vi "Dielectric vs Temperature - freq (4284A).vi"() -> ()   [LabVIEW 2010]
uses:
  <vilib>/Instr/_visa.llb/VISA Configure Serial Port (Instr).vi
  Instance          14 32Saved   K vs Temp - freq (4284A) .vi
  Instance          13 32Saved   K vs Temp - freq (4284A) .vi
  Instance          12 32Saved   K vs Temp - freq (4284A) .vi
  Instance          11 32Saved   K vs Temp - freq (4284A) .vi
  Instance          26 32Saved   K vs Temp - freq (4284A) .vi
  Instance          25 32Saved   K vs Temp - freq (4284A) .vi
  Instance          10 32Saved   K vs Temp - freq (4284A) .vi
  Instance           9 32Saved   K vs Temp - freq (4284A) .vi
  Instance           8 32Saved   K vs Temp - freq (4284A) .vi
  Instance           7 32Saved   K vs Temp - freq (4284A) .vi
  Instance          24 32Saved   K vs Temp - freq (4284A) .vi
  Instance          22 32Saved   K vs Temp - freq (4284A) .vi
  Instance          20 32Saved   K vs Temp - freq (4284A) .vi
  Instance          18 32Saved   K vs Temp - freq (4284A) .vi
  Instance          23 32Saved   K vs Temp - freq (4284A) .vi
  Instance          21 32Saved   K vs Temp - freq (4284A) .vi
  Instance          19 32Saved   K vs Temp - freq (4284A) .vi
  Instance          17 32Saved   K vs Temp - freq (4284A) .vi
  Instance          16 32Saved   K vs Temp - freq (4284A) .vi
  Instance          15 32Saved   K vs Temp - freq (4284A) .vi
  Instance           6 32Saved   K vs Temp - freq (4284A) .vi
  Instance           5 32Saved   K vs Temp - freq (4284A) .vi
  <vilib>/Utility/file.llb/Write To Spreadsheet File (DBL).vi
panel:
  in  "Freq Value (Hz) (1MHz)":dbl=1000000.0
  out "tand1M":dbl
  out "K1M":dbl
  out "C1M":dbl
  out "Temp1MHz":dbl format="%#_3g"
  in  "Freq Value (Hz) (500kHz)":dbl=500000.0
  out "tand500k":dbl
  out "K500k":dbl
  out "C500k":dbl
  out "Temp500kHz":dbl format="%#_3g"
  in  "Freq Value (Hz) (250kHz)":dbl=250000.0
  out "tand250k":dbl
  out "K250k":dbl
  out "C250k":dbl
  out "Temp250kHz":dbl format="%#_3g"
  in  "Freq Value (Hz) (100kHz)":dbl=100000.0
  out "tand100k":dbl
  out "K100k":dbl
  out "C100k":dbl
  out "Temp100kHz":dbl format="%#_3g"
  in  "Freq Value (Hz) (50kHz)":dbl=50000.0
  out "tand50k":dbl
  out "K50k":dbl
  out "C50k":dbl
  out "Temp50kHz":dbl format="%#_3g"
  in  "Freq Value (Hz) (25kHz)":dbl=25000.0
  out "tand25k":dbl
  out "K25k":dbl
  out "C25k":dbl
  out "Temp25kHz":dbl format="%#_3g"
  in  "Freq Value (Hz) (10kHz)":dbl=10000.0
  out "tand10k":dbl
  out "K10k":dbl
  out "C10k":dbl
  out "Temp10kHz":dbl format="%#_3g"
  in  "Freq Value (Hz) (5kHz)":dbl=5000.0
  out "tand5k":dbl
  out "K5k":dbl
  out "C5k":dbl
  out "Temp5kHz":dbl format="%#_3g"
  in  "Freq Value (Hz) (2.5kHz)":dbl=2500.0
  out "tand2.5k":dbl
  out "K2.5k":dbl
  out "C2.5k":dbl
  out "Temp2.5kHz":dbl format="%#_3g"
  in  "Freq Value (Hz) (1kHz)":dbl=1000.0
  out "tand1k":dbl
  out "K1k":dbl
  out "C1k":dbl
  out "Temp1kHz":dbl format="%#_3g"
  in  "tand500k":dbl[](array[numeric])
  in  "K500k":dbl[](array[numeric])
  in  "Temp500k":dbl[](array[numeric])
  out "Temp500Hz":dbl format="%#_3g"
  out "C500":dbl
  out "?":dbl
  out "tand500":dbl
  in  "Freq Value (Hz) (500Hz)":dbl=500.0
  in  "Freq Value (Hz) (250Hz)":dbl=250.0
  in  "Freq Value (Hz) (100Hz)":dbl=100.0
  in  "Freq Value (Hz) (50Hz)":dbl=50.0
  in  "Freq Value (Hz) (25Hz)":dbl=25.0
  in  "tand100k":dbl[](array[numeric])
  in  "tand10k":dbl[](array[numeric])
  in  "tand1k":dbl[](array[numeric])
  in  "tand100":dbl[](array[numeric])
  in  "K100k":dbl[](array[numeric])
  in  "K10k":dbl[](array[numeric])
  in  "K1k":dbl[](array[numeric])
  in  "K100":dbl[](array[numeric])
  in  "Temp100k":dbl[](array[numeric])
  in  "Temp10k":dbl[](array[numeric])
  in  "Temp1k":dbl[](array[numeric])
  in  "Temp100":dbl[](array[numeric])
  out "Temp250Hz":dbl format="%#_3g"
  out "Temp100Hz":dbl format="%#_3g"
  out "tand25":dbl
  out "Temp50Hz":dbl format="%#_3g"
  in  "VISA Omega (Serial - COM1)":refnum<visa-resource-name>
  in  "VISA Agilent 4284A (GPIB)":refnum<visa-resource-name>
  in  "Run":bool
  out "Thickness":dbl
  out "Area":dbl
  in  "stop":bool
  out "tand250":dbl
  out "tand100":dbl
  out "tand50":dbl
  out "K250":dbl
  out "K100":dbl
  out "K50":dbl
  out "K25":dbl
  out "C250":dbl
  out "C100":dbl
  out "C50":dbl
  out "C25":dbl
  out "Temp25Hz":dbl format="%#_3g"
  out "Dielectric Loss vs. Temperature":cluster{"Y":dbl[], "Y":dbl[]}[](graph)
  out "Relative Permittivity vs. Temperature":cluster{"Y":dbl[], "Y":dbl[]}[](graph)
  in  "Comment (Sample's Name, compositions, whatever you want,..)":string
  in  "Thickness (mm)":dbl
  in  "Diameter (mm)":dbl
  in  "Path & File Name (*.txt)":path
  # "Temperature (C)"
  # "Frequency (Hz)"
  # "Capacitance (F)"
  # "Relative Permittivity"
  # "Dielectric Loss"
  # "Sample Details"
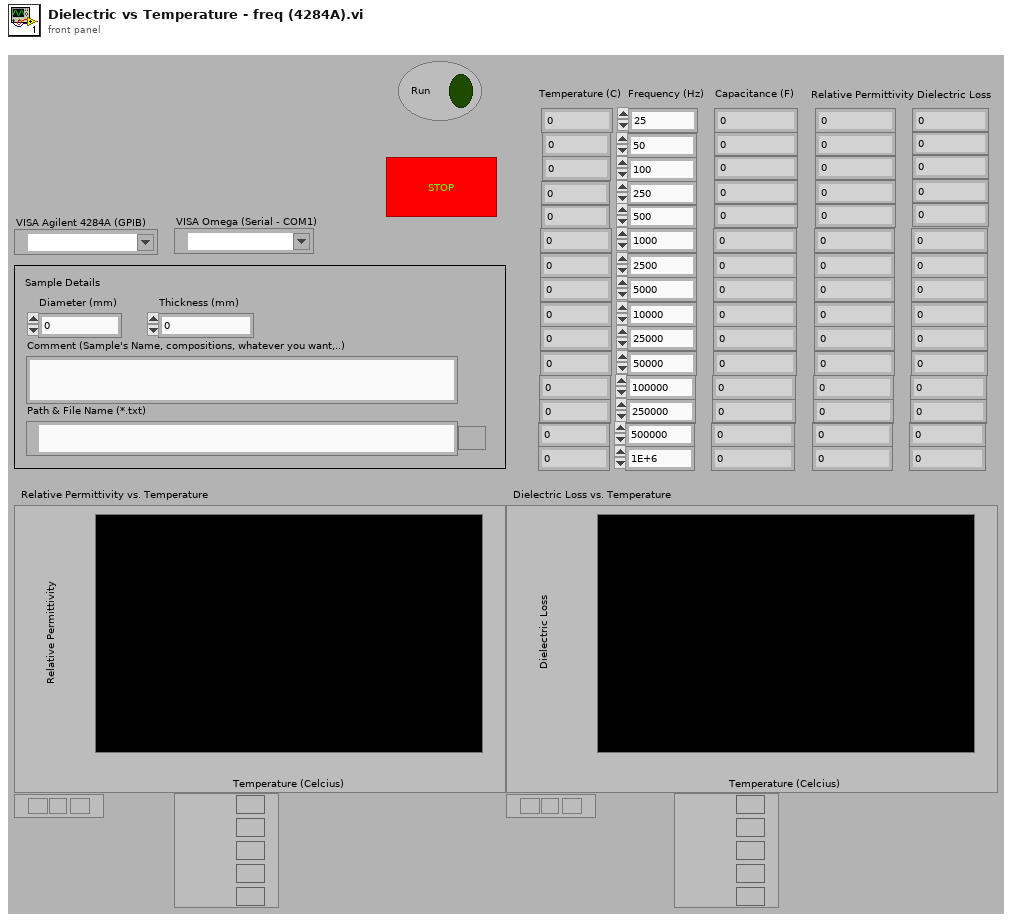
[diagram p1: front panel]
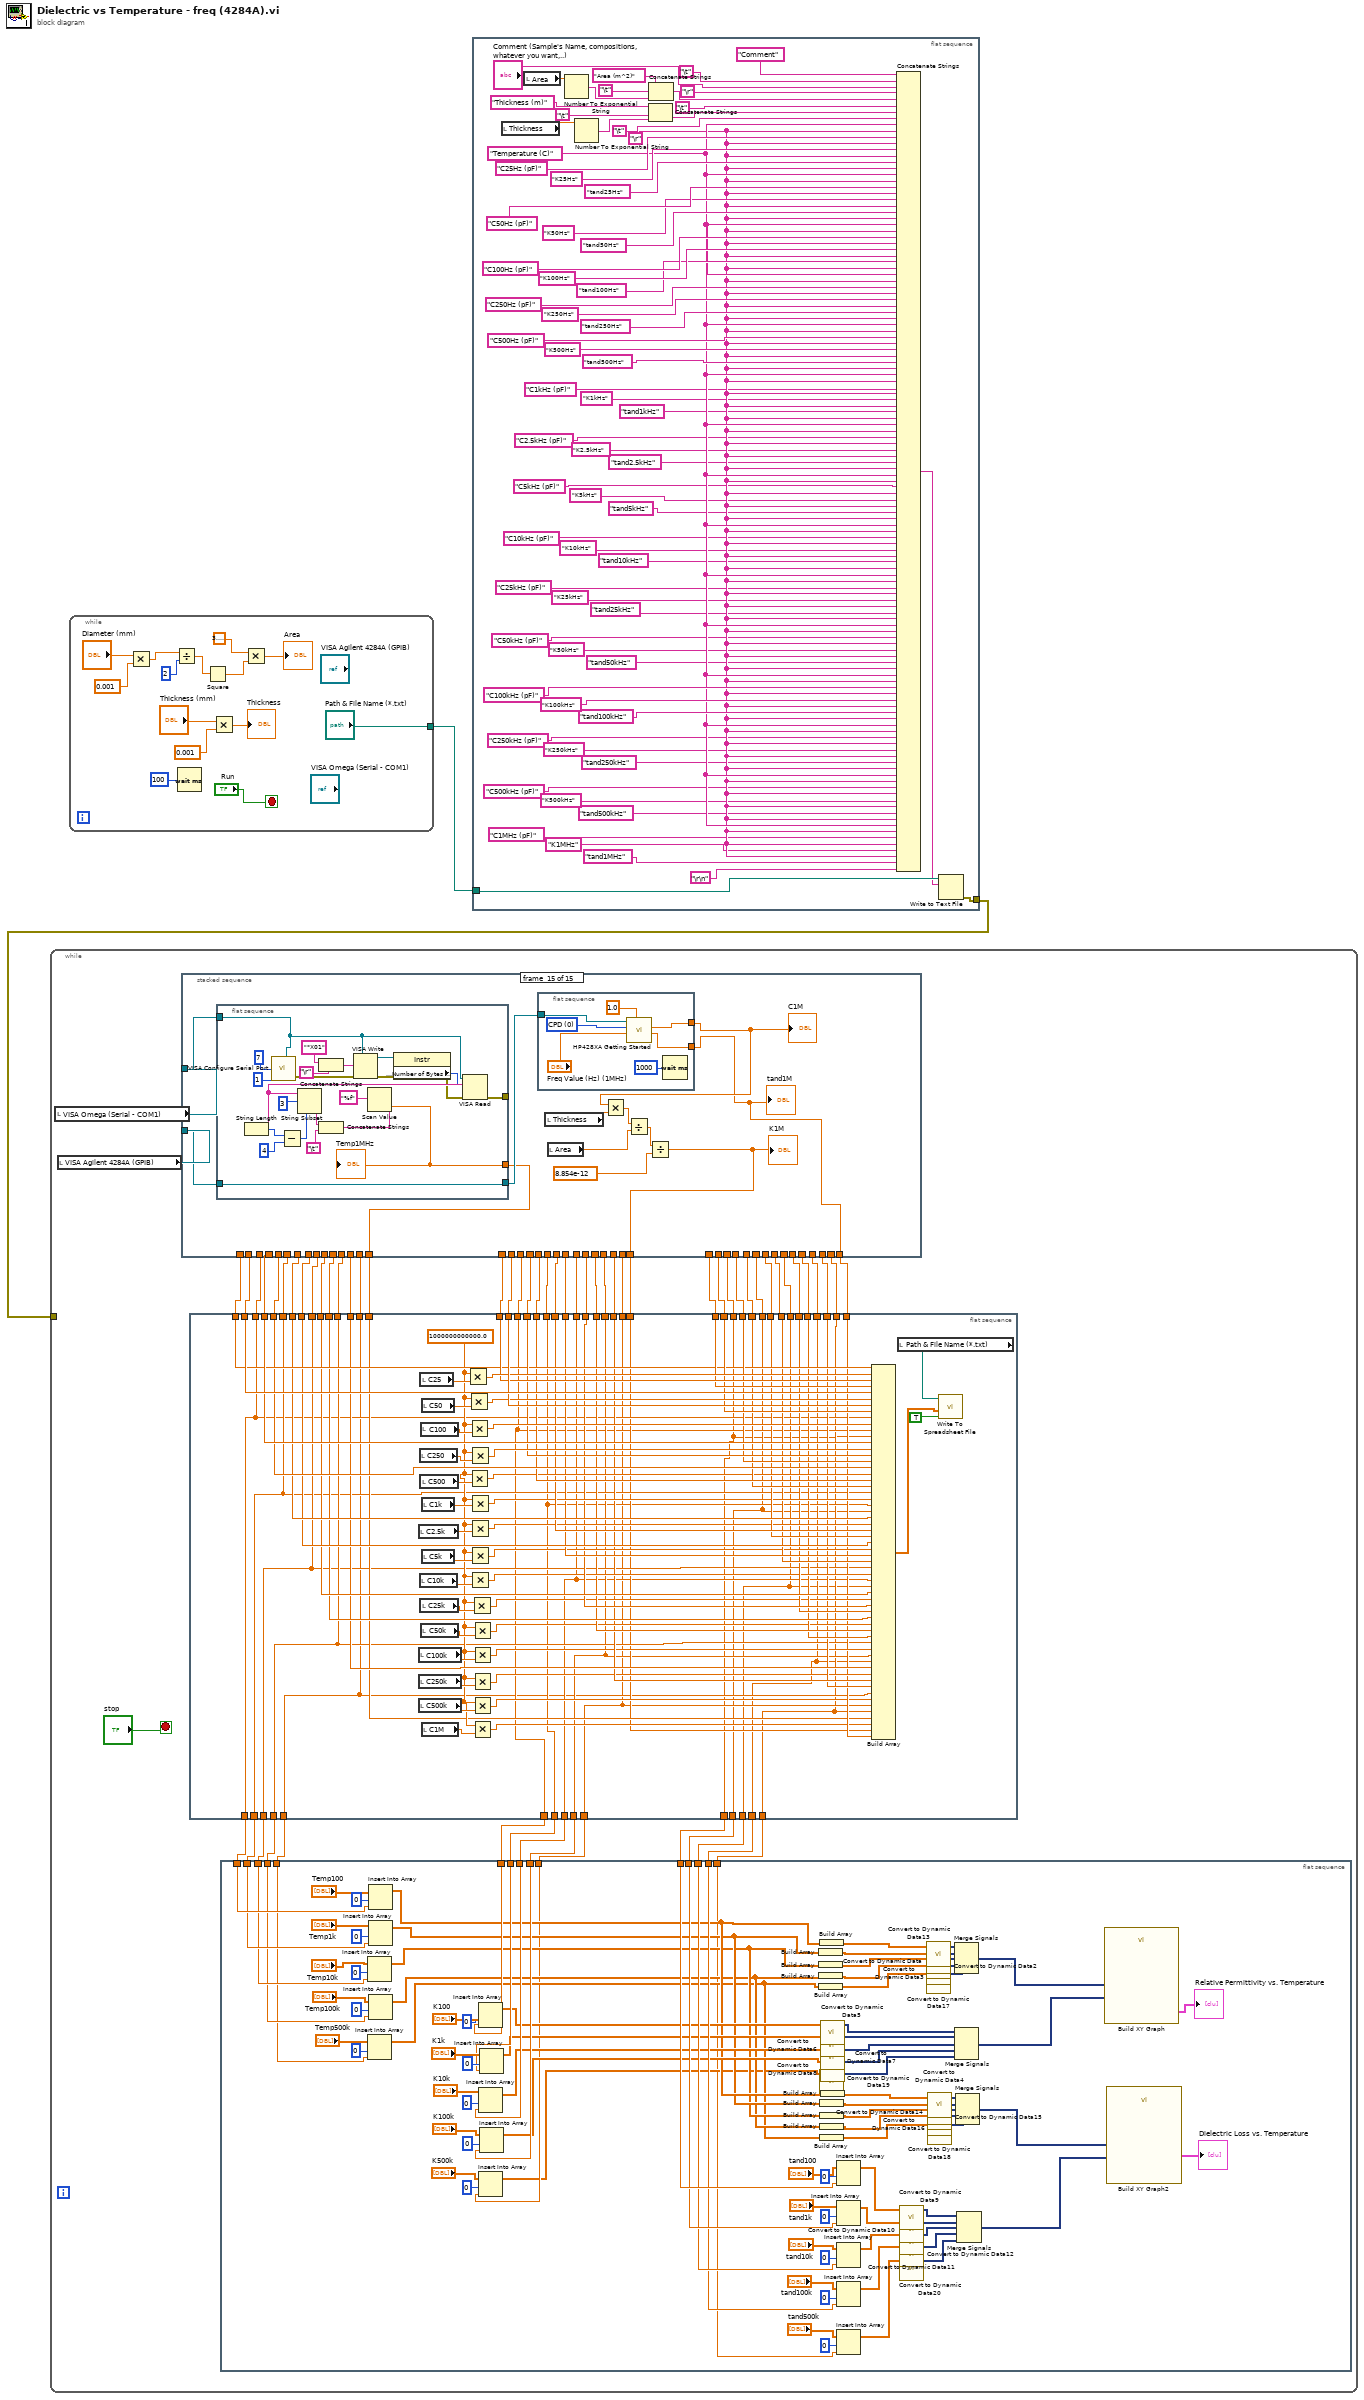
[diagram p0: block diagram]
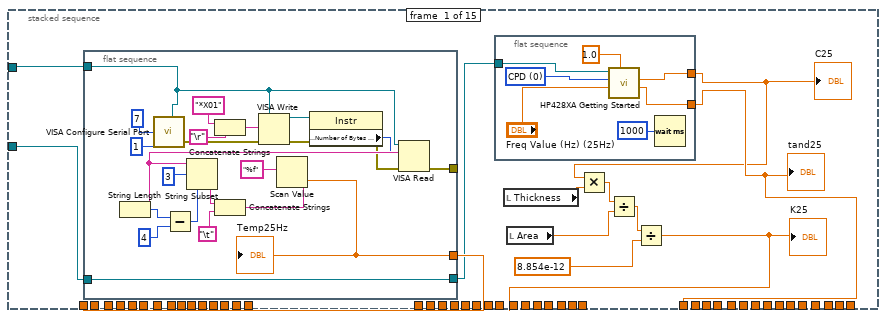
[diagram p2: hidden frame]
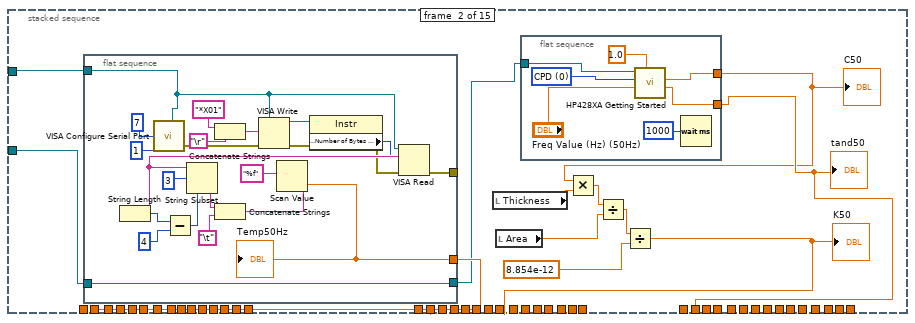
[diagram p3: hidden frame]
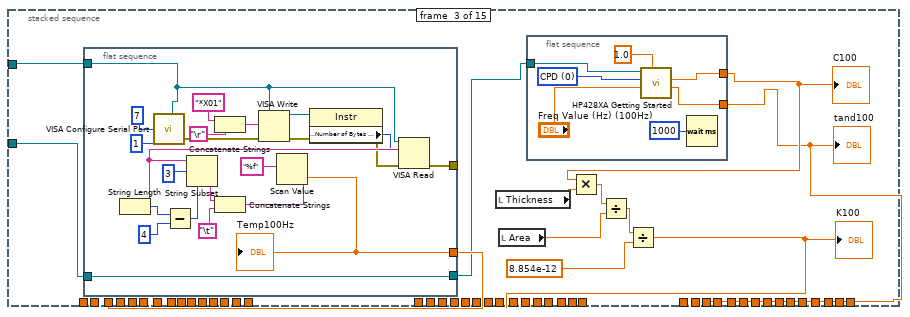
[diagram p4: hidden frame]
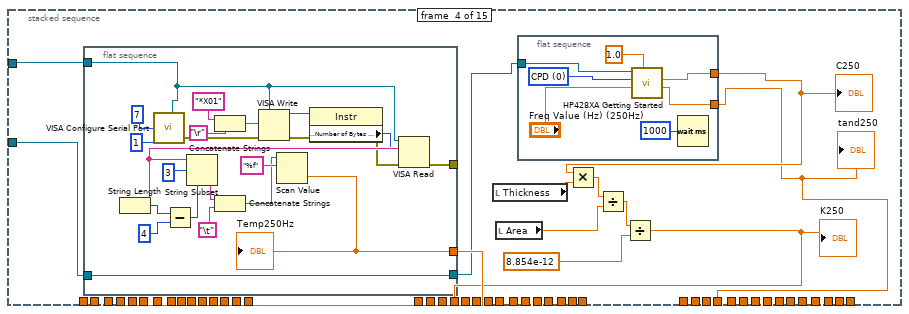
[diagram p5: hidden frame]
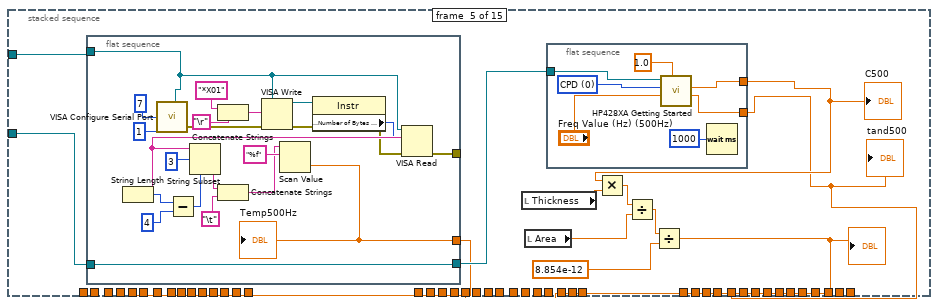
[diagram p6: hidden frame]
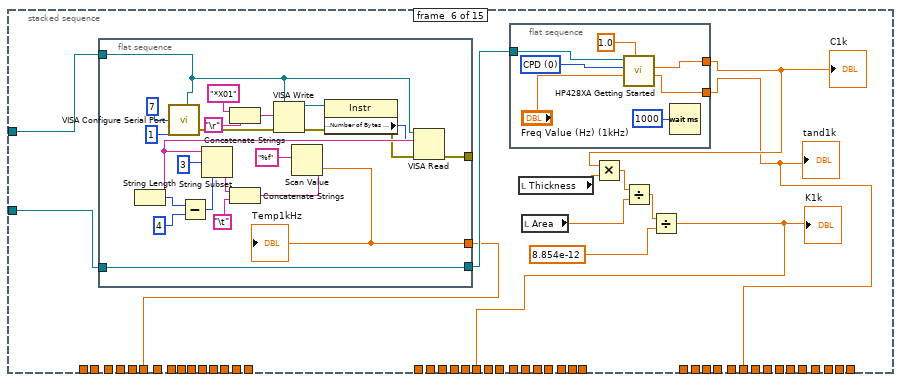
[diagram p7: hidden frame]
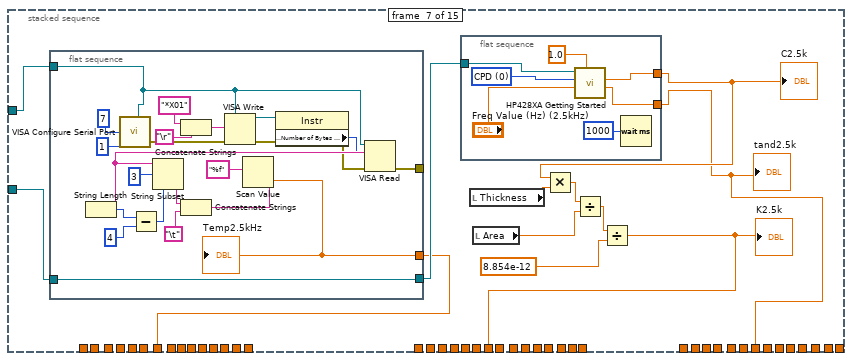
[diagram p8: hidden frame]
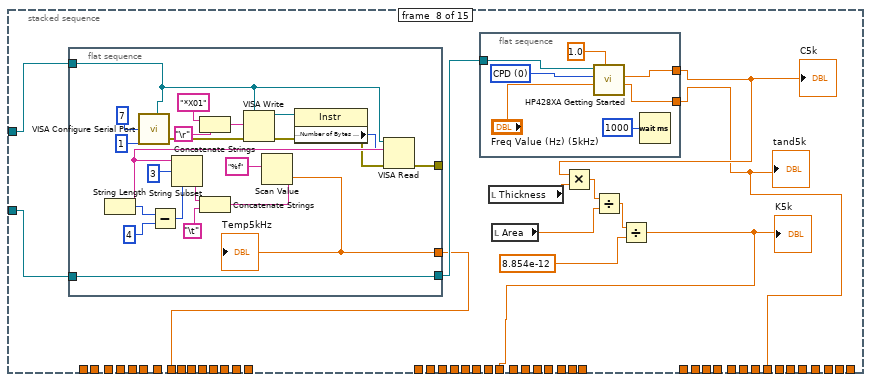
[diagram p9: hidden frame]
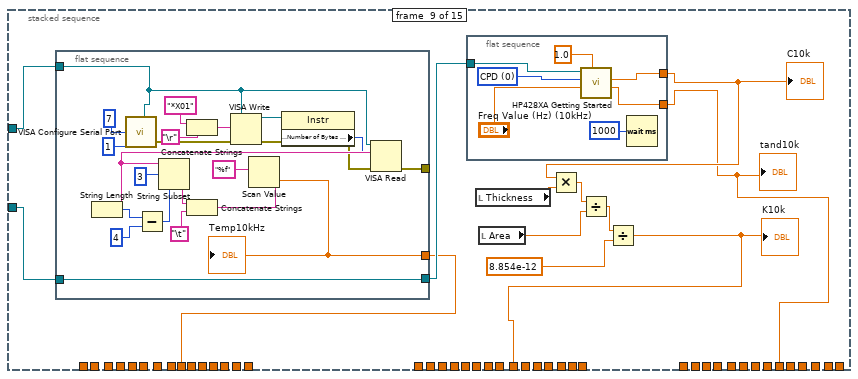
[diagram p10: hidden frame]
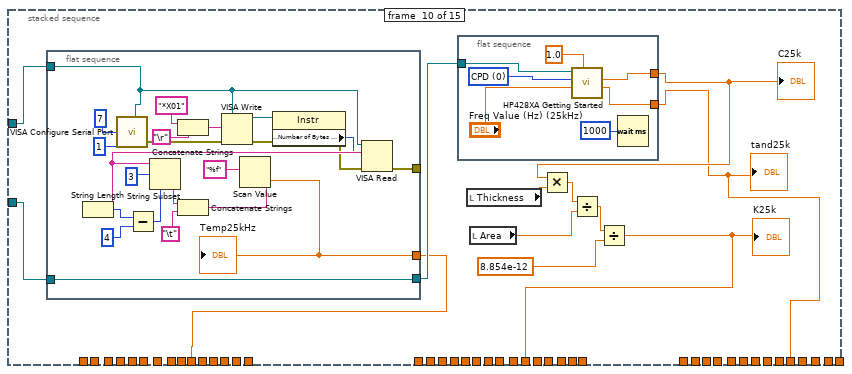
[diagram p11: hidden frame]
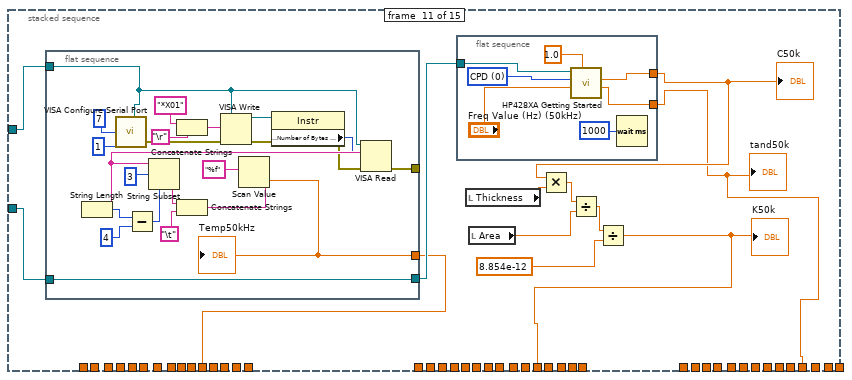
[diagram p12: hidden frame]
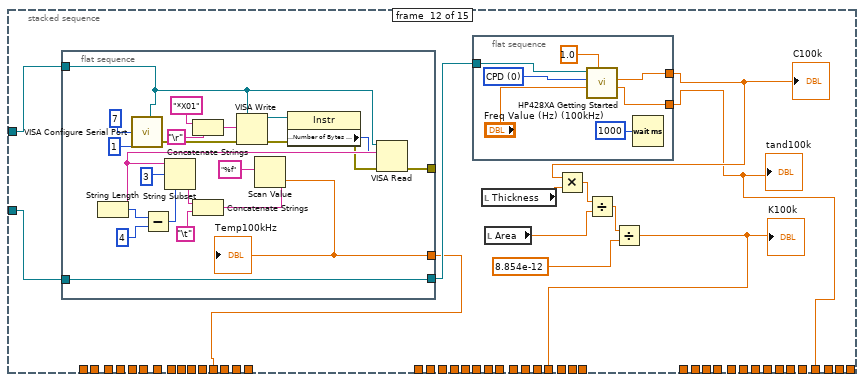
[diagram p13: hidden frame]
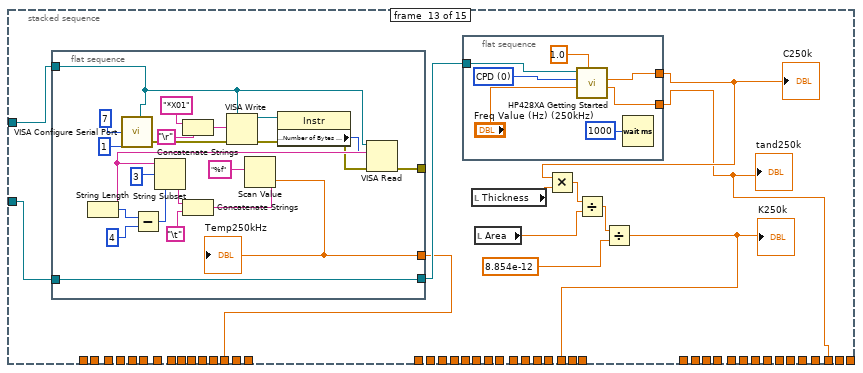
[diagram p14: hidden frame]
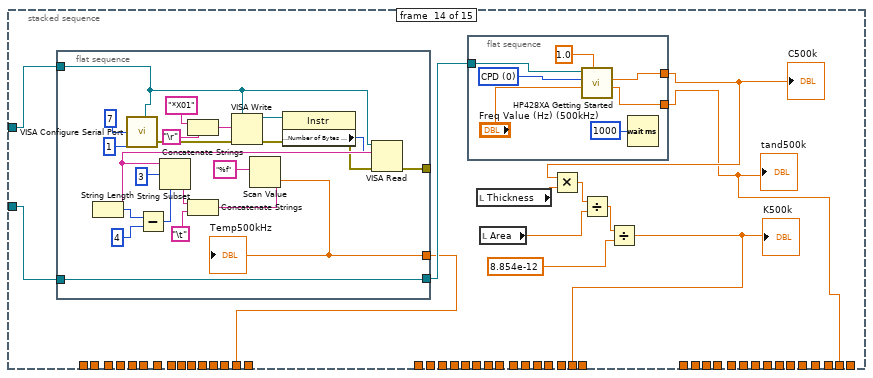
[diagram p15: hidden frame]
diagram:
  n1 = while {
    tunnel: w1 -> [_]
    stop <- "stop" stop-if-true
    n2 = local read "VISA Omega (Serial - COM1)"() -> (w52:refnum<visa-resource-name>)
    n3 = local read "VISA Agilent 4284A (GPIB)"() -> (w51:refnum<visa-resource-name>)
    n4 = stacked-sequence {
      tunnel: w52 -> [w252 w294 w336 w378 w413 w455 w497 w539 w581 w623 w665 w707 w749 w791 w833]
      tunnel: w51 -> [w251 w293 w335 w377 w414 w454 w496 w538 w580 w622 w664 w706 w748 w790 w832]
      tunnel: [w245 _ _ _ _ _ _ _ _ _ _ _ _ _ _] -> w53
      tunnel: [_ w287 _ _ _ _ _ _ _ _ _ _ _ _ _] -> w64
      tunnel: [_ _ w329 _ _ _ _ _ _ _ _ _ _ _ _] -> w63
      tunnel: [_ _ _ w371 _ _ _ _ _ _ _ _ _ _ _] -> w62
      tunnel: [w244 _ _ _ _ _ _ _ _ _ _ _ _ _ _] -> w61
      tunnel: [_ w286 _ _ _ _ _ _ _ _ _ _ _ _ _] -> w60
      tunnel: [_ _ w328 _ _ _ _ _ _ _ _ _ _ _ _] -> w59
      tunnel: [_ _ _ w370 _ _ _ _ _ _ _ _ _ _ _] -> w58
      tunnel: [w242 _ _ _ _ _ _ _ _ _ _ _ _ _ _] -> w57
      tunnel: [_ w285 _ _ _ _ _ _ _ _ _ _ _ _ _] -> w56
      tunnel: [_ _ w325 _ _ _ _ _ _ _ _ _ _ _ _] -> w55
      tunnel: [_ _ _ w367 _ _ _ _ _ _ _ _ _ _ _] -> w54
      tunnel: [_ _ _ _ w411 _ _ _ _ _ _ _ _ _ _] -> w50
      tunnel: [_ _ _ _ w410 _ _ _ _ _ _ _ _ _ _] -> w49
      tunnel: [_ _ _ _ w409 _ _ _ _ _ _ _ _ _ _] -> w48
      tunnel: [_ _ _ _ _ w453 _ _ _ _ _ _ _ _ _] -> w47
      tunnel: [_ _ _ _ _ w452 _ _ _ _ _ _ _ _ _] -> w46
      tunnel: [_ _ _ _ _ w451 _ _ _ _ _ _ _ _ _] -> w45
      tunnel: [_ _ _ _ _ _ w495 _ _ _ _ _ _ _ _] -> w44
      tunnel: [_ _ _ _ _ _ w494 _ _ _ _ _ _ _ _] -> w43
      tunnel: [_ _ _ _ _ _ w493 _ _ _ _ _ _ _ _] -> w42
      tunnel: [_ _ _ _ _ _ _ w537 _ _ _ _ _ _ _] -> w41
      tunnel: [_ _ _ _ _ _ _ w536 _ _ _ _ _ _ _] -> w40
      tunnel: [_ _ _ _ _ _ _ w535 _ _ _ _ _ _ _] -> w39
      tunnel: [_ _ _ _ _ _ _ _ w579 _ _ _ _ _ _] -> w38
      tunnel: [_ _ _ _ _ _ _ _ w578 _ _ _ _ _ _] -> w37
      tunnel: [_ _ _ _ _ _ _ _ w577 _ _ _ _ _ _] -> w36
      tunnel: [_ _ _ _ _ _ _ _ _ w621 _ _ _ _ _] -> w35
      tunnel: [_ _ _ _ _ _ _ _ _ w620 _ _ _ _ _] -> w34
      tunnel: [_ _ _ _ _ _ _ _ _ w619 _ _ _ _ _] -> w33
      tunnel: [_ _ _ _ _ _ _ _ _ _ w663 _ _ _ _] -> w32
      tunnel: [_ _ _ _ _ _ _ _ _ _ w662 _ _ _ _] -> w31
      tunnel: [_ _ _ _ _ _ _ _ _ _ w661 _ _ _ _] -> w30
      tunnel: [_ _ _ _ _ _ _ _ _ _ _ w705 _ _ _] -> w29
      tunnel: [_ _ _ _ _ _ _ _ _ _ _ w704 _ _ _] -> w28
      tunnel: [_ _ _ _ _ _ _ _ _ _ _ w703 _ _ _] -> w27
      tunnel: [_ _ _ _ _ _ _ _ _ _ _ _ w747 _ _] -> w26
      tunnel: [_ _ _ _ _ _ _ _ _ _ _ _ w746 _ _] -> w25
      tunnel: [_ _ _ _ _ _ _ _ _ _ _ _ w745 _ _] -> w24
      tunnel: [_ _ _ _ _ _ _ _ _ _ _ _ _ w789 _] -> w23
      tunnel: [_ _ _ _ _ _ _ _ _ _ _ _ _ w788 _] -> w22
      tunnel: [_ _ _ _ _ _ _ _ _ _ _ _ _ w787 _] -> w21
      tunnel: [_ _ _ _ _ _ _ _ _ _ _ _ _ _ w831] -> w18
      tunnel: [_ _ _ _ _ _ _ _ _ _ _ _ _ _ w830] -> w19
      tunnel: [_ _ _ _ _ _ _ _ _ _ _ _ _ _ w829] -> w20
      frame #0 {
        n5 = flat-sequence {
          tunnel: w252 -> [w263]
          tunnel: [w262] -> _
          tunnel: [w261] -> w245
          tunnel: w251 -> [w260]
          tunnel: [w260] -> w243
          frame #0 {
            n6 = call-poly "VISA Configure Serial Port"("VISA resource name"=w263, "data bits (8)"=7, "parity (0:none)"=1) -> ("error out"=w268:errorcluster)  [unwired: 11 in, 1 out]
            n7 = Concatenate Strings("*X01", "\r") -> (w271:string)
            n8 = VISA Write(VISA resource name=w263, write buffer=w271, error in (no error)=w268) -> (VISA resource name out=w282:refnum<visa-resource-name>, error out=w272:errorcluster)  [unwired: 1 out]
            n9 = property class="Instr"(reference=w282, error in=w272) -> (error out=w273:errorcluster, "Serial Settings:Number of Bytes at Serial Port"=w274:u32)  [unwired: 1 out]
            n10 = VISA Read(VISA resource name=w263, byte count=w274, error in (no error)=w273) -> (read buffer=w275:string, error out=w262:errorcluster)  [unwired: 2 out]
            n11 = String Length(string=w275) -> (length=w277:i32)
            n12 = Subtract(x=w277, y=4) -> (x-y=w279:i32)
            n13 = String Subset(string=w275, offset (0)=3, length (rest)=w279) -> (substring=w280:string)
            n14 = Concatenate Strings(w280, "\t") -> (w264:string)
            n15 = Scan Value(string=w264, format string="%f") -> (value=w261:dbl)  [unwired: 1 in, 1 out]
            "Temp25Hz" <- w261
          }
        }
        n16 = flat-sequence {
          tunnel: w243 -> [w258]
          tunnel: [w255] -> w242
          tunnel: [w254] -> w241
          frame #0 {
            w257 = u32 0 items=["CPD", "CPQ", "CPG", "CPRP", "CSD", "CSQ", "CSRS", "LPQ", "LPD", "LPG", "LPRP", "LSD", "LSQ", "LSRS", "RX", "ZTD", "ZTR", "GB", "YTD", "YTR"] ("Imp Type (0: CPD)")
            n17 = call "HP428XA Getting Started.vi"("Voltage Level (V) (1.0V)"=1.0, "Freq Value (Hz) (1.0 MHz)"="Freq Value (Hz) (25Hz)", "Imp Type (0: CPD)"=w257, "GPIB Address (15)"=w258) -> ("Secondary Value"=w255:dbl, "Primary Value"=w254:dbl)  [unwired: 4 in, 2 out]
            n18 = Wait (ms)(milliseconds to wait=u32 1000) -> ()  [unwired: 1 out]
          }
        }
        n19 = local read "Thickness"() -> (w250:dbl)
        n20 = local read "Area"() -> (w248:dbl)
        n21 = Multiply(x=w241, y=w250) -> (x*y=w249:dbl)
        n22 = Divide(x=w249, y=w248) -> (x/y=w247:dbl)
        n23 = Divide(x=w247, y=8.854e-12) -> (x/y=w244:dbl)
        "K25" <- w244
        "C25" <- w241
        "tand25" <- w242
      }
      frame #1 {
        n24 = flat-sequence {
          tunnel: w294 -> [w305]
          tunnel: [w304] -> _
          tunnel: [w303] -> w287
          tunnel: w293 -> [w302]
          tunnel: [w302] -> w283
          frame #0 {
            n25 = call-poly "VISA Configure Serial Port"("VISA resource name"=w305, "data bits (8)"=7, "parity (0:none)"=1) -> ("error out"=w310:errorcluster)  [unwired: 11 in, 1 out]
            n26 = Concatenate Strings("*X01", "\r") -> (w313:string)
            n27 = VISA Write(VISA resource name=w305, write buffer=w313, error in (no error)=w310) -> (VISA resource name out=w324:refnum<visa-resource-name>, error out=w314:errorcluster)  [unwired: 1 out]
            n28 = property class="Instr"(reference=w324, error in=w314) -> (error out=w315:errorcluster, "Serial Settings:Number of Bytes at Serial Port"=w316:u32)  [unwired: 1 out]
            n29 = VISA Read(VISA resource name=w305, byte count=w316, error in (no error)=w315) -> (read buffer=w317:string, error out=w304:errorcluster)  [unwired: 2 out]
            n30 = String Length(string=w317) -> (length=w319:i32)
            n31 = Subtract(x=w319, y=4) -> (x-y=w321:i32)
            n32 = String Subset(string=w317, offset (0)=3, length (rest)=w321) -> (substring=w322:string)
            n33 = Concatenate Strings(w322, "\t") -> (w306:string)
            n34 = Scan Value(string=w306, format string="%f") -> (value=w303:dbl)  [unwired: 1 in, 1 out]
            "Temp50Hz" <- w303
          }
        }
        n35 = local read "Thickness"() -> (w292:dbl)
        n36 = local read "Area"() -> (w290:dbl)
        n37 = flat-sequence {
          tunnel: w283 -> [w300]
          tunnel: [w297] -> w285
          tunnel: [w296] -> w284
          frame #0 {
            w299 = u32 0 items=["CPD", "CPQ", "CPG", "CPRP", "CSD", "CSQ", "CSRS", "LPQ", "LPD", "LPG", "LPRP", "LSD", "LSQ", "LSRS", "RX", "ZTD", "ZTR", "GB", "YTD", "YTR"] ("Imp Type (0: CPD)")
            n38 = call "HP428XA Getting Started.vi"("Voltage Level (V) (1.0V)"=1.0, "Freq Value (Hz) (1.0 MHz)"="Freq Value (Hz) (50Hz)", "Imp Type (0: CPD)"=w299, "GPIB Address (15)"=w300) -> ("Secondary Value"=w297:dbl, "Primary Value"=w296:dbl)  [unwired: 4 in, 2 out]
            n39 = Wait (ms)(milliseconds to wait=u32 1000) -> ()  [unwired: 1 out]
          }
        }
        n40 = Multiply(x=w284, y=w292) -> (x*y=w291:dbl)
        n41 = Divide(x=w291, y=w290) -> (x/y=w289:dbl)
        n42 = Divide(x=w289, y=8.854e-12) -> (x/y=w286:dbl)
        "K50" <- w286
        "tand50" <- w285
        "C50" <- w284
      }
      frame #2 {
        n43 = flat-sequence {
          tunnel: w336 -> [w347]
          tunnel: [w346] -> _
          tunnel: [w345] -> w329
          tunnel: w335 -> [w344]
          tunnel: [w344] -> w327
          frame #0 {
            n44 = call-poly "VISA Configure Serial Port"("VISA resource name"=w347, "data bits (8)"=7, "parity (0:none)"=1) -> ("error out"=w352:errorcluster)  [unwired: 11 in, 1 out]
            n45 = Concatenate Strings("*X01", "\r") -> (w355:string)
            n46 = VISA Write(VISA resource name=w347, write buffer=w355, error in (no error)=w352) -> (VISA resource name out=w366:refnum<visa-resource-name>, error out=w356:errorcluster)  [unwired: 1 out]
            n47 = property class="Instr"(reference=w366, error in=w356) -> (error out=w357:errorcluster, "Serial Settings:Number of Bytes at Serial Port"=w358:u32)  [unwired: 1 out]
            n48 = VISA Read(VISA resource name=w347, byte count=w358, error in (no error)=w357) -> (read buffer=w359:string, error out=w346:errorcluster)  [unwired: 2 out]
            n49 = String Length(string=w359) -> (length=w361:i32)
            n50 = Subtract(x=w361, y=4) -> (x-y=w363:i32)
            n51 = String Subset(string=w359, offset (0)=3, length (rest)=w363) -> (substring=w364:string)
            n52 = Concatenate Strings(w364, "\t") -> (w348:string)
            n53 = Scan Value(string=w348, format string="%f") -> (value=w345:dbl)  [unwired: 1 in, 1 out]
            "Temp100Hz" <- w345
          }
        }
        n54 = local read "Thickness"() -> (w334:dbl)
        n55 = local read "Area"() -> (w332:dbl)
        n56 = flat-sequence {
          tunnel: w327 -> [w342]
          tunnel: [w339] -> w325
          tunnel: [w338] -> w326
          frame #0 {
            w341 = u32 0 items=["CPD", "CPQ", "CPG", "CPRP", "CSD", "CSQ", "CSRS", "LPQ", "LPD", "LPG", "LPRP", "LSD", "LSQ", "LSRS", "RX", "ZTD", "ZTR", "GB", "YTD", "YTR"] ("Imp Type (0: CPD)")
            n57 = call "HP428XA Getting Started.vi"("Voltage Level (V) (1.0V)"=1.0, "Freq Value (Hz) (1.0 MHz)"="Freq Value (Hz) (100Hz)", "Imp Type (0: CPD)"=w341, "GPIB Address (15)"=w342) -> ("Secondary Value"=w339:dbl, "Primary Value"=w338:dbl)  [unwired: 4 in, 2 out]
            n58 = Wait (ms)(milliseconds to wait=u32 1000) -> ()  [unwired: 1 out]
          }
        }
        n59 = Multiply(x=w326, y=w334) -> (x*y=w333:dbl)
        n60 = Divide(x=w333, y=w332) -> (x/y=w331:dbl)
        n61 = Divide(x=w331, y=8.854e-12) -> (x/y=w328:dbl)
        "K100" <- w328
        "C100" <- w326
        "tand100" <- w325
      }
      frame #3 {
        n62 = flat-sequence {
          tunnel: w378 -> [w389]
          tunnel: [w388] -> _
          tunnel: [w387] -> w371
          tunnel: w377 -> [w386]
          tunnel: [w386] -> w369
          frame #0 {
            n63 = call-poly "VISA Configure Serial Port"("VISA resource name"=w389, "data bits (8)"=7, "parity (0:none)"=1) -> ("error out"=w394:errorcluster)  [unwired: 11 in, 1 out]
            n64 = Concatenate Strings("*X01", "\r") -> (w397:string)
            n65 = VISA Write(VISA resource name=w389, write buffer=w397, error in (no error)=w394) -> (VISA resource name out=w408:refnum<visa-resource-name>, error out=w398:errorcluster)  [unwired: 1 out]
            n66 = property class="Instr"(reference=w408, error in=w398) -> (error out=w399:errorcluster, "Serial Settings:Number of Bytes at Serial Port"=w400:u32)  [unwired: 1 out]
            n67 = VISA Read(VISA resource name=w389, byte count=w400, error in (no error)=w399) -> (read buffer=w401:string, error out=w388:errorcluster)  [unwired: 2 out]
            n68 = String Length(string=w401) -> (length=w403:i32)
            n69 = Subtract(x=w403, y=4) -> (x-y=w405:i32)
            n70 = String Subset(string=w401, offset (0)=3, length (rest)=w405) -> (substring=w406:string)
            n71 = Concatenate Strings(w406, "\t") -> (w390:string)
            n72 = Scan Value(string=w390, format string="%f") -> (value=w387:dbl)  [unwired: 1 in, 1 out]
            "Temp250Hz" <- w387
          }
        }
        n73 = local read "Thickness"() -> (w376:dbl)
        n74 = local read "Area"() -> (w374:dbl)
        n75 = flat-sequence {
          tunnel: w369 -> [w384]
          tunnel: [w381] -> w367
          tunnel: [w380] -> w368
          frame #0 {
            w383 = u32 0 items=["CPD", "CPQ", "CPG", "CPRP", "CSD", "CSQ", "CSRS", "LPQ", "LPD", "LPG", "LPRP", "LSD", "LSQ", "LSRS", "RX", "ZTD", "ZTR", "GB", "YTD", "YTR"] ("Imp Type (0: CPD)")
            n76 = call "HP428XA Getting Started.vi"("Voltage Level (V) (1.0V)"=1.0, "Freq Value (Hz) (1.0 MHz)"="Freq Value (Hz) (250Hz)", "Imp Type (0: CPD)"=w383, "GPIB Address (15)"=w384) -> ("Secondary Value"=w381:dbl, "Primary Value"=w380:dbl)  [unwired: 4 in, 2 out]
            n77 = Wait (ms)(milliseconds to wait=u32 1000) -> ()  [unwired: 1 out]
          }
        }
        n78 = Multiply(x=w368, y=w376) -> (x*y=w375:dbl)
        n79 = Divide(x=w375, y=w374) -> (x/y=w373:dbl)
        n80 = Divide(x=w373, y=8.854e-12) -> (x/y=w370:dbl)
        "K250" <- w370
        "C250" <- w368
        "tand250" <- w367
      }
      frame #4 {
        n81 = flat-sequence {
          tunnel: w413 -> [w431]
          tunnel: [w430] -> _
          tunnel: [w429] -> w411
          tunnel: w414 -> [w428]
          tunnel: [w428] -> w412
          frame #0 {
            n82 = call-poly "VISA Configure Serial Port"("VISA resource name"=w431, "data bits (8)"=7, "parity (0:none)"=1) -> ("error out"=w436:errorcluster)  [unwired: 11 in, 1 out]
            n83 = Concatenate Strings("*X01", "\r") -> (w439:string)
            n84 = VISA Write(VISA resource name=w431, write buffer=w439, error in (no error)=w436) -> (VISA resource name out=w450:refnum<visa-resource-name>, error out=w440:errorcluster)  [unwired: 1 out]
            n85 = property class="Instr"(reference=w450, error in=w440) -> (error out=w441:errorcluster, "Serial Settings:Number of Bytes at Serial Port"=w442:u32)  [unwired: 1 out]
            n86 = VISA Read(VISA resource name=w431, byte count=w442, error in (no error)=w441) -> (read buffer=w443:string, error out=w430:errorcluster)  [unwired: 2 out]
            n87 = String Length(string=w443) -> (length=w445:i32)
            n88 = Subtract(x=w445, y=4) -> (x-y=w447:i32)
            n89 = String Subset(string=w443, offset (0)=3, length (rest)=w447) -> (substring=w448:string)
            n90 = Concatenate Strings(w448, "\t") -> (w432:string)
            n91 = Scan Value(string=w432, format string="%f") -> (value=w429:dbl)  [unwired: 1 in, 1 out]
            "Temp500Hz" <- w429
          }
        }
        n92 = local read "Thickness"() -> (w420:dbl)
        n93 = local read "Area"() -> (w418:dbl)
        n94 = flat-sequence {
          tunnel: w412 -> [w426]
          tunnel: [w423] -> w409
          tunnel: [w422] -> w415
          frame #0 {
            w425 = u32 0 items=["CPD", "CPQ", "CPG", "CPRP", "CSD", "CSQ", "CSRS", "LPQ", "LPD", "LPG", "LPRP", "LSD", "LSQ", "LSRS", "RX", "ZTD", "ZTR", "GB", "YTD", "YTR"] ("Imp Type (0: CPD)")
            n95 = call "HP428XA Getting Started.vi"("Voltage Level (V) (1.0V)"=1.0, "Freq Value (Hz) (1.0 MHz)"="Freq Value (Hz) (500Hz)", "Imp Type (0: CPD)"=w425, "GPIB Address (15)"=w426) -> ("Secondary Value"=w423:dbl, "Primary Value"=w422:dbl)  [unwired: 4 in, 2 out]
            n96 = Wait (ms)(milliseconds to wait=u32 1000) -> ()  [unwired: 1 out]
          }
        }
        n97 = Multiply(x=w415, y=w420) -> (x*y=w419:dbl)
        n98 = Divide(x=w419, y=w418) -> (x/y=w417:dbl)
        n99 = Divide(x=w417, y=8.854e-12) -> (x/y=w410:dbl)
        "?" <- w410
        "C500" <- w415
        "tand500" <- w409
      }
      frame #5 {
        n100 = flat-sequence {
          tunnel: w455 -> [w473]
          tunnel: [w472] -> _
          tunnel: [w471] -> w453
          tunnel: w454 -> [w470]
          tunnel: [w470] -> w457
          frame #0 {
            n101 = call-poly "VISA Configure Serial Port"("VISA resource name"=w473, "data bits (8)"=7, "parity (0:none)"=1) -> ("error out"=w478:errorcluster)  [unwired: 11 in, 1 out]
            n102 = Concatenate Strings("*X01", "\r") -> (w481:string)
            n103 = VISA Write(VISA resource name=w473, write buffer=w481, error in (no error)=w478) -> (VISA resource name out=w492:refnum<visa-resource-name>, error out=w482:errorcluster)  [unwired: 1 out]
            n104 = property class="Instr"(reference=w492, error in=w482) -> (error out=w483:errorcluster, "Serial Settings:Number of Bytes at Serial Port"=w484:u32)  [unwired: 1 out]
            n105 = VISA Read(VISA resource name=w473, byte count=w484, error in (no error)=w483) -> (read buffer=w485:string, error out=w472:errorcluster)  [unwired: 2 out]
            n106 = String Length(string=w485) -> (length=w487:i32)
            n107 = Subtract(x=w487, y=4) -> (x-y=w489:i32)
            n108 = String Subset(string=w485, offset (0)=3, length (rest)=w489) -> (substring=w490:string)
            n109 = Concatenate Strings(w490, "\t") -> (w474:string)
            n110 = Scan Value(string=w474, format string="%f") -> (value=w471:dbl)  [unwired: 1 in, 1 out]
            "Temp1kHz" <- w471
          }
        }
        n111 = flat-sequence {
          tunnel: w457 -> [w468]
          tunnel: [w465] -> w451
          tunnel: [w464] -> w456
          frame #0 {
            w467 = u32 0 items=["CPD", "CPQ", "CPG", "CPRP", "CSD", "CSQ", "CSRS", "LPQ", "LPD", "LPG", "LPRP", "LSD", "LSQ", "LSRS", "RX", "ZTD", "ZTR", "GB", "YTD", "YTR"] ("Imp Type (0: CPD)")
            n112 = call "HP428XA Getting Started.vi"("Voltage Level (V) (1.0V)"=1.0, "Freq Value (Hz) (1.0 MHz)"="Freq Value (Hz) (1kHz)", "Imp Type (0: CPD)"=w467, "GPIB Address (15)"=w468) -> ("Secondary Value"=w465:dbl, "Primary Value"=w464:dbl)  [unwired: 4 in, 2 out]
            n113 = Wait (ms)(milliseconds to wait=u32 1000) -> ()  [unwired: 1 out]
          }
        }
        n114 = local read "Thickness"() -> (w462:dbl)
        n115 = local read "Area"() -> (w460:dbl)
        n116 = Multiply(x=w456, y=w462) -> (x*y=w461:dbl)
        n117 = Divide(x=w461, y=w460) -> (x/y=w459:dbl)
        n118 = Divide(x=w459, y=8.854e-12) -> (x/y=w452:dbl)
        "K1k" <- w452
        "C1k" <- w456
        "tand1k" <- w451
      }
      frame #6 {
        n119 = flat-sequence {
          tunnel: w497 -> [w515]
          tunnel: [w514] -> _
          tunnel: [w513] -> w495
          tunnel: w496 -> [w512]
          tunnel: [w512] -> w499
          frame #0 {
            n120 = call-poly "VISA Configure Serial Port"("VISA resource name"=w515, "data bits (8)"=7, "parity (0:none)"=1) -> ("error out"=w520:errorcluster)  [unwired: 11 in, 1 out]
            n121 = Concatenate Strings("*X01", "\r") -> (w523:string)
            n122 = VISA Write(VISA resource name=w515, write buffer=w523, error in (no error)=w520) -> (VISA resource name out=w534:refnum<visa-resource-name>, error out=w524:errorcluster)  [unwired: 1 out]
            n123 = property class="Instr"(reference=w534, error in=w524) -> (error out=w525:errorcluster, "Serial Settings:Number of Bytes at Serial Port"=w526:u32)  [unwired: 1 out]
            n124 = VISA Read(VISA resource name=w515, byte count=w526, error in (no error)=w525) -> (read buffer=w527:string, error out=w514:errorcluster)  [unwired: 2 out]
            n125 = String Length(string=w527) -> (length=w529:i32)
            n126 = Subtract(x=w529, y=4) -> (x-y=w531:i32)
            n127 = String Subset(string=w527, offset (0)=3, length (rest)=w531) -> (substring=w532:string)
            n128 = Concatenate Strings(w532, "\t") -> (w516:string)
            n129 = Scan Value(string=w516, format string="%f") -> (value=w513:dbl)  [unwired: 1 in, 1 out]
            "Temp2.5kHz" <- w513
          }
        }
        n130 = flat-sequence {
          tunnel: w499 -> [w510]
          tunnel: [w507] -> w493
          tunnel: [w506] -> w498
          frame #0 {
            w509 = u32 0 items=["CPD", "CPQ", "CPG", "CPRP", "CSD", "CSQ", "CSRS", "LPQ", "LPD", "LPG", "LPRP", "LSD", "LSQ", "LSRS", "RX", "ZTD", "ZTR", "GB", "YTD", "YTR"] ("Imp Type (0: CPD)")
            n131 = call "HP428XA Getting Started.vi"("Voltage Level (V) (1.0V)"=1.0, "Freq Value (Hz) (1.0 MHz)"="Freq Value (Hz) (2.5kHz)", "Imp Type (0: CPD)"=w509, "GPIB Address (15)"=w510) -> ("Secondary Value"=w507:dbl, "Primary Value"=w506:dbl)  [unwired: 4 in, 2 out]
            n132 = Wait (ms)(milliseconds to wait=u32 1000) -> ()  [unwired: 1 out]
          }
        }
        n133 = local read "Thickness"() -> (w504:dbl)
        n134 = local read "Area"() -> (w502:dbl)
        n135 = Multiply(x=w498, y=w504) -> (x*y=w503:dbl)
        n136 = Divide(x=w503, y=w502) -> (x/y=w501:dbl)
        n137 = Divide(x=w501, y=8.854e-12) -> (x/y=w494:dbl)
        "K2.5k" <- w494
        "C2.5k" <- w498
        "tand2.5k" <- w493
      }
      frame #7 {
        n138 = flat-sequence {
          tunnel: w539 -> [w557]
          tunnel: [w556] -> _
          tunnel: [w555] -> w537
          tunnel: w538 -> [w554]
          tunnel: [w554] -> w541
          frame #0 {
            n139 = call-poly "VISA Configure Serial Port"("VISA resource name"=w557, "data bits (8)"=7, "parity (0:none)"=1) -> ("error out"=w562:errorcluster)  [unwired: 11 in, 1 out]
            n140 = Concatenate Strings("*X01", "\r") -> (w565:string)
            n141 = VISA Write(VISA resource name=w557, write buffer=w565, error in (no error)=w562) -> (VISA resource name out=w576:refnum<visa-resource-name>, error out=w566:errorcluster)  [unwired: 1 out]
            n142 = property class="Instr"(reference=w576, error in=w566) -> (error out=w567:errorcluster, "Serial Settings:Number of Bytes at Serial Port"=w568:u32)  [unwired: 1 out]
            n143 = VISA Read(VISA resource name=w557, byte count=w568, error in (no error)=w567) -> (read buffer=w569:string, error out=w556:errorcluster)  [unwired: 2 out]
            n144 = String Length(string=w569) -> (length=w571:i32)
            n145 = Subtract(x=w571, y=4) -> (x-y=w573:i32)
            n146 = String Subset(string=w569, offset (0)=3, length (rest)=w573) -> (substring=w574:string)
            n147 = Concatenate Strings(w574, "\t") -> (w558:string)
            n148 = Scan Value(string=w558, format string="%f") -> (value=w555:dbl)  [unwired: 1 in, 1 out]
            "Temp5kHz" <- w555
          }
        }
        n149 = flat-sequence {
          tunnel: w541 -> [w552]
          tunnel: [w549] -> w535
          tunnel: [w548] -> w540
          frame #0 {
            w551 = u32 0 items=["CPD", "CPQ", "CPG", "CPRP", "CSD", "CSQ", "CSRS", "LPQ", "LPD", "LPG", "LPRP", "LSD", "LSQ", "LSRS", "RX", "ZTD", "ZTR", "GB", "YTD", "YTR"] ("Imp Type (0: CPD)")
            n150 = call "HP428XA Getting Started.vi"("Voltage Level (V) (1.0V)"=1.0, "Freq Value (Hz) (1.0 MHz)"="Freq Value (Hz) (5kHz)", "Imp Type (0: CPD)"=w551, "GPIB Address (15)"=w552) -> ("Secondary Value"=w549:dbl, "Primary Value"=w548:dbl)  [unwired: 4 in, 2 out]
            n151 = Wait (ms)(milliseconds to wait=u32 1000) -> ()  [unwired: 1 out]
          }
        }
        n152 = local read "Thickness"() -> (w546:dbl)
        n153 = local read "Area"() -> (w544:dbl)
        n154 = Multiply(x=w540, y=w546) -> (x*y=w545:dbl)
        n155 = Divide(x=w545, y=w544) -> (x/y=w543:dbl)
        n156 = Divide(x=w543, y=8.854e-12) -> (x/y=w536:dbl)
        "K5k" <- w536
        "C5k" <- w540
        "tand5k" <- w535
      }
      frame #8 {
        n157 = flat-sequence {
          tunnel: w581 -> [w599]
          tunnel: [w598] -> _
          tunnel: [w597] -> w579
          tunnel: w580 -> [w596]
          tunnel: [w596] -> w583
          frame #0 {
            n158 = call-poly "VISA Configure Serial Port"("VISA resource name"=w599, "data bits (8)"=7, "parity (0:none)"=1) -> ("error out"=w604:errorcluster)  [unwired: 11 in, 1 out]
            n159 = Concatenate Strings("*X01", "\r") -> (w607:string)
            n160 = VISA Write(VISA resource name=w599, write buffer=w607, error in (no error)=w604) -> (VISA resource name out=w618:refnum<visa-resource-name>, error out=w608:errorcluster)  [unwired: 1 out]
            n161 = property class="Instr"(reference=w618, error in=w608) -> (error out=w609:errorcluster, "Serial Settings:Number of Bytes at Serial Port"=w610:u32)  [unwired: 1 out]
            n162 = VISA Read(VISA resource name=w599, byte count=w610, error in (no error)=w609) -> (read buffer=w611:string, error out=w598:errorcluster)  [unwired: 2 out]
            n163 = String Length(string=w611) -> (length=w613:i32)
            n164 = Subtract(x=w613, y=4) -> (x-y=w615:i32)
            n165 = String Subset(string=w611, offset (0)=3, length (rest)=w615) -> (substring=w616:string)
            n166 = Concatenate Strings(w616, "\t") -> (w600:string)
            n167 = Scan Value(string=w600, format string="%f") -> (value=w597:dbl)  [unwired: 1 in, 1 out]
            "Temp10kHz" <- w597
          }
        }
        n168 = flat-sequence {
          tunnel: w583 -> [w594]
          tunnel: [w591] -> w577
          tunnel: [w590] -> w582
          frame #0 {
            w593 = u32 0 items=["CPD", "CPQ", "CPG", "CPRP", "CSD", "CSQ", "CSRS", "LPQ", "LPD", "LPG", "LPRP", "LSD", "LSQ", "LSRS", "RX", "ZTD", "ZTR", "GB", "YTD", "YTR"] ("Imp Type (0: CPD)")
            n169 = call "HP428XA Getting Started.vi"("Voltage Level (V) (1.0V)"=1.0, "Freq Value (Hz) (1.0 MHz)"="Freq Value (Hz) (10kHz)", "Imp Type (0: CPD)"=w593, "GPIB Address (15)"=w594) -> ("Secondary Value"=w591:dbl, "Primary Value"=w590:dbl)  [unwired: 4 in, 2 out]
            n170 = Wait (ms)(milliseconds to wait=u32 1000) -> ()  [unwired: 1 out]
          }
        }
        n171 = local read "Thickness"() -> (w588:dbl)
        n172 = local read "Area"() -> (w586:dbl)
        n173 = Multiply(x=w582, y=w588) -> (x*y=w587:dbl)
        n174 = Divide(x=w587, y=w586) -> (x/y=w585:dbl)
        n175 = Divide(x=w585, y=8.854e-12) -> (x/y=w578:dbl)
        "K10k" <- w578
        "C10k" <- w582
        "tand10k" <- w577
      }
      frame #9 {
        n176 = flat-sequence {
          tunnel: w623 -> [w641]
          tunnel: [w640] -> _
          tunnel: [w639] -> w621
          tunnel: w622 -> [w638]
          tunnel: [w638] -> w625
          frame #0 {
            n177 = call-poly "VISA Configure Serial Port"("VISA resource name"=w641, "data bits (8)"=7, "parity (0:none)"=1) -> ("error out"=w646:errorcluster)  [unwired: 11 in, 1 out]
            n178 = Concatenate Strings("*X01", "\r") -> (w649:string)
            n179 = VISA Write(VISA resource name=w641, write buffer=w649, error in (no error)=w646) -> (VISA resource name out=w660:refnum<visa-resource-name>, error out=w650:errorcluster)  [unwired: 1 out]
            n180 = property class="Instr"(reference=w660, error in=w650) -> (error out=w651:errorcluster, "Serial Settings:Number of Bytes at Serial Port"=w652:u32)  [unwired: 1 out]
            n181 = VISA Read(VISA resource name=w641, byte count=w652, error in (no error)=w651) -> (read buffer=w653:string, error out=w640:errorcluster)  [unwired: 2 out]
            n182 = String Length(string=w653) -> (length=w655:i32)
            n183 = Subtract(x=w655, y=4) -> (x-y=w657:i32)
            n184 = String Subset(string=w653, offset (0)=3, length (rest)=w657) -> (substring=w658:string)
            n185 = Concatenate Strings(w658, "\t") -> (w642:string)
            n186 = Scan Value(string=w642, format string="%f") -> (value=w639:dbl)  [unwired: 1 in, 1 out]
            "Temp25kHz" <- w639
          }
        }
        n187 = flat-sequence {
          tunnel: w625 -> [w636]
          tunnel: [w633] -> w619
          tunnel: [w632] -> w624
          frame #0 {
            w635 = u32 0 items=["CPD", "CPQ", "CPG", "CPRP", "CSD", "CSQ", "CSRS", "LPQ", "LPD", "LPG", "LPRP", "LSD", "LSQ", "LSRS", "RX", "ZTD", "ZTR", "GB", "YTD", "YTR"] ("Imp Type (0: CPD)")
            n188 = call "HP428XA Getting Started.vi"("Voltage Level (V) (1.0V)"=1.0, "Freq Value (Hz) (1.0 MHz)"="Freq Value (Hz) (25kHz)", "Imp Type (0: CPD)"=w635, "GPIB Address (15)"=w636) -> ("Secondary Value"=w633:dbl, "Primary Value"=w632:dbl)  [unwired: 4 in, 2 out]
            n189 = Wait (ms)(milliseconds to wait=u32 1000) -> ()  [unwired: 1 out]
          }
        }
        n190 = local read "Thickness"() -> (w630:dbl)
        n191 = local read "Area"() -> (w628:dbl)
        n192 = Multiply(x=w624, y=w630) -> (x*y=w629:dbl)
        n193 = Divide(x=w629, y=w628) -> (x/y=w627:dbl)
        n194 = Divide(x=w627, y=8.854e-12) -> (x/y=w620:dbl)
        "K25k" <- w620
        "C25k" <- w624
        "tand25k" <- w619
      }
      frame #10 {
        n195 = flat-sequence {
          tunnel: w665 -> [w683]
          tunnel: [w682] -> _
          tunnel: [w681] -> w663
          tunnel: w664 -> [w680]
          tunnel: [w680] -> w667
          frame #0 {
            n196 = call-poly "VISA Configure Serial Port"("VISA resource name"=w683, "data bits (8)"=7, "parity (0:none)"=1) -> ("error out"=w688:errorcluster)  [unwired: 11 in, 1 out]
            n197 = Concatenate Strings("*X01", "\r") -> (w691:string)
            n198 = VISA Write(VISA resource name=w683, write buffer=w691, error in (no error)=w688) -> (VISA resource name out=w702:refnum<visa-resource-name>, error out=w692:errorcluster)  [unwired: 1 out]
            n199 = property class="Instr"(reference=w702, error in=w692) -> (error out=w693:errorcluster, "Serial Settings:Number of Bytes at Serial Port"=w694:u32)  [unwired: 1 out]
            n200 = VISA Read(VISA resource name=w683, byte count=w694, error in (no error)=w693) -> (read buffer=w695:string, error out=w682:errorcluster)  [unwired: 2 out]
            n201 = String Length(string=w695) -> (length=w697:i32)
            n202 = Subtract(x=w697, y=4) -> (x-y=w699:i32)
            n203 = String Subset(string=w695, offset (0)=3, length (rest)=w699) -> (substring=w700:string)
            n204 = Concatenate Strings(w700, "\t") -> (w684:string)
            n205 = Scan Value(string=w684, format string="%f") -> (value=w681:dbl)  [unwired: 1 in, 1 out]
            "Temp50kHz" <- w681
          }
        }
        n206 = flat-sequence {
          tunnel: w667 -> [w678]
          tunnel: [w675] -> w661
          tunnel: [w674] -> w666
          frame #0 {
            w677 = u32 0 items=["CPD", "CPQ", "CPG", "CPRP", "CSD", "CSQ", "CSRS", "LPQ", "LPD", "LPG", "LPRP", "LSD", "LSQ", "LSRS", "RX", "ZTD", "ZTR", "GB", "YTD", "YTR"] ("Imp Type (0: CPD)")
            n207 = call "HP428XA Getting Started.vi"("Voltage Level (V) (1.0V)"=1.0, "Freq Value (Hz) (1.0 MHz)"="Freq Value (Hz) (50kHz)", "Imp Type (0: CPD)"=w677, "GPIB Address (15)"=w678) -> ("Secondary Value"=w675:dbl, "Primary Value"=w674:dbl)  [unwired: 4 in, 2 out]
            n208 = Wait (ms)(milliseconds to wait=u32 1000) -> ()  [unwired: 1 out]
          }
        }
        n209 = local read "Thickness"() -> (w672:dbl)
        n210 = local read "Area"() -> (w670:dbl)
        n211 = Multiply(x=w666, y=w672) -> (x*y=w671:dbl)
        n212 = Divide(x=w671, y=w670) -> (x/y=w669:dbl)
        n213 = Divide(x=w669, y=8.854e-12) -> (x/y=w662:dbl)
        "K50k" <- w662
        "C50k" <- w666
        "tand50k" <- w661
      }
      frame #11 {
        n214 = flat-sequence {
          tunnel: w707 -> [w725]
          tunnel: [w724] -> _
          tunnel: [w723] -> w705
          tunnel: w706 -> [w722]
          tunnel: [w722] -> w709
          frame #0 {
            n215 = call-poly "VISA Configure Serial Port"("VISA resource name"=w725, "data bits (8)"=7, "parity (0:none)"=1) -> ("error out"=w730:errorcluster)  [unwired: 11 in, 1 out]
            n216 = Concatenate Strings("*X01", "\r") -> (w733:string)
            n217 = VISA Write(VISA resource name=w725, write buffer=w733, error in (no error)=w730) -> (VISA resource name out=w744:refnum<visa-resource-name>, error out=w734:errorcluster)  [unwired: 1 out]
            n218 = property class="Instr"(reference=w744, error in=w734) -> (error out=w735:errorcluster, "Serial Settings:Number of Bytes at Serial Port"=w736:u32)  [unwired: 1 out]
            n219 = VISA Read(VISA resource name=w725, byte count=w736, error in (no error)=w735) -> (read buffer=w737:string, error out=w724:errorcluster)  [unwired: 2 out]
            n220 = String Length(string=w737) -> (length=w739:i32)
            n221 = Subtract(x=w739, y=4) -> (x-y=w741:i32)
            n222 = String Subset(string=w737, offset (0)=3, length (rest)=w741) -> (substring=w742:string)
            n223 = Concatenate Strings(w742, "\t") -> (w726:string)
            n224 = Scan Value(string=w726, format string="%f") -> (value=w723:dbl)  [unwired: 1 in, 1 out]
            "Temp100kHz" <- w723
          }
        }
        n225 = flat-sequence {
          tunnel: w709 -> [w720]
          tunnel: [w717] -> w703
          tunnel: [w716] -> w708
          frame #0 {
            w719 = u32 0 items=["CPD", "CPQ", "CPG", "CPRP", "CSD", "CSQ", "CSRS", "LPQ", "LPD", "LPG", "LPRP", "LSD", "LSQ", "LSRS", "RX", "ZTD", "ZTR", "GB", "YTD", "YTR"] ("Imp Type (0: CPD)")
            n226 = call "HP428XA Getting Started.vi"("Voltage Level (V) (1.0V)"=1.0, "Freq Value (Hz) (1.0 MHz)"="Freq Value (Hz) (100kHz)", "Imp Type (0: CPD)"=w719, "GPIB Address (15)"=w720) -> ("Secondary Value"=w717:dbl, "Primary Value"=w716:dbl)  [unwired: 4 in, 2 out]
            n227 = Wait (ms)(milliseconds to wait=u32 1000) -> ()  [unwired: 1 out]
          }
        }
        n228 = local read "Thickness"() -> (w714:dbl)
        n229 = local read "Area"() -> (w712:dbl)
        n230 = Multiply(x=w708, y=w714) -> (x*y=w713:dbl)
        n231 = Divide(x=w713, y=w712) -> (x/y=w711:dbl)
        n232 = Divide(x=w711, y=8.854e-12) -> (x/y=w704:dbl)
        "K100k" <- w704
        "C100k" <- w708
        "tand100k" <- w703
      }
      frame #12 {
        n233 = flat-sequence {
          tunnel: w749 -> [w767]
          tunnel: [w766] -> _
          tunnel: [w765] -> w747
          tunnel: w748 -> [w764]
          tunnel: [w764] -> w751
          frame #0 {
            n234 = call-poly "VISA Configure Serial Port"("VISA resource name"=w767, "data bits (8)"=7, "parity (0:none)"=1) -> ("error out"=w772:errorcluster)  [unwired: 11 in, 1 out]
            n235 = Concatenate Strings("*X01", "\r") -> (w775:string)
            n236 = VISA Write(VISA resource name=w767, write buffer=w775, error in (no error)=w772) -> (VISA resource name out=w786:refnum<visa-resource-name>, error out=w776:errorcluster)  [unwired: 1 out]
            n237 = property class="Instr"(reference=w786, error in=w776) -> (error out=w777:errorcluster, "Serial Settings:Number of Bytes at Serial Port"=w778:u32)  [unwired: 1 out]
            n238 = VISA Read(VISA resource name=w767, byte count=w778, error in (no error)=w777) -> (read buffer=w779:string, error out=w766:errorcluster)  [unwired: 2 out]
            n239 = String Length(string=w779) -> (length=w781:i32)
            n240 = Subtract(x=w781, y=4) -> (x-y=w783:i32)
            n241 = String Subset(string=w779, offset (0)=3, length (rest)=w783) -> (substring=w784:string)
            n242 = Concatenate Strings(w784, "\t") -> (w768:string)
            n243 = Scan Value(string=w768, format string="%f") -> (value=w765:dbl)  [unwired: 1 in, 1 out]
            "Temp250kHz" <- w765
          }
        }
        n244 = flat-sequence {
          tunnel: w751 -> [w762]
          tunnel: [w759] -> w745
          tunnel: [w758] -> w750
          frame #0 {
            w761 = u32 0 items=["CPD", "CPQ", "CPG", "CPRP", "CSD", "CSQ", "CSRS", "LPQ", "LPD", "LPG", "LPRP", "LSD", "LSQ", "LSRS", "RX", "ZTD", "ZTR", "GB", "YTD", "YTR"] ("Imp Type (0: CPD)")
            n245 = call "HP428XA Getting Started.vi"("Voltage Level (V) (1.0V)"=1.0, "Freq Value (Hz) (1.0 MHz)"="Freq Value (Hz) (250kHz)", "Imp Type (0: CPD)"=w761, "GPIB Address (15)"=w762) -> ("Secondary Value"=w759:dbl, "Primary Value"=w758:dbl)  [unwired: 4 in, 2 out]
            n246 = Wait (ms)(milliseconds to wait=u32 1000) -> ()  [unwired: 1 out]
          }
        }
        n247 = local read "Thickness"() -> (w756:dbl)
        n248 = local read "Area"() -> (w754:dbl)
        n249 = Multiply(x=w750, y=w756) -> (x*y=w755:dbl)
        n250 = Divide(x=w755, y=w754) -> (x/y=w753:dbl)
        n251 = Divide(x=w753, y=8.854e-12) -> (x/y=w746:dbl)
        "K250k" <- w746
        "C250k" <- w750
        "tand250k" <- w745
      }
      frame #13 {
        n252 = flat-sequence {
          tunnel: w791 -> [w809]
          tunnel: [w808] -> _
          tunnel: [w807] -> w789
          tunnel: w790 -> [w806]
          tunnel: [w806] -> w793
          frame #0 {
            n253 = call-poly "VISA Configure Serial Port"("VISA resource name"=w809, "data bits (8)"=7, "parity (0:none)"=1) -> ("error out"=w814:errorcluster)  [unwired: 11 in, 1 out]
            n254 = Concatenate Strings("*X01", "\r") -> (w817:string)
            n255 = VISA Write(VISA resource name=w809, write buffer=w817, error in (no error)=w814) -> (VISA resource name out=w828:refnum<visa-resource-name>, error out=w818:errorcluster)  [unwired: 1 out]
            n256 = property class="Instr"(reference=w828, error in=w818) -> (error out=w819:errorcluster, "Serial Settings:Number of Bytes at Serial Port"=w820:u32)  [unwired: 1 out]
            n257 = VISA Read(VISA resource name=w809, byte count=w820, error in (no error)=w819) -> (read buffer=w821:string, error out=w808:errorcluster)  [unwired: 2 out]
            n258 = String Length(string=w821) -> (length=w823:i32)
            n259 = Subtract(x=w823, y=4) -> (x-y=w825:i32)
            n260 = String Subset(string=w821, offset (0)=3, length (rest)=w825) -> (substring=w826:string)
            n261 = Concatenate Strings(w826, "\t") -> (w810:string)
            n262 = Scan Value(string=w810, format string="%f") -> (value=w807:dbl)  [unwired: 1 in, 1 out]
            "Temp500kHz" <- w807
          }
        }
        n263 = flat-sequence {
          tunnel: w793 -> [w804]
          tunnel: [w801] -> w787
          tunnel: [w800] -> w792
          frame #0 {
            w803 = u32 0 items=["CPD", "CPQ", "CPG", "CPRP", "CSD", "CSQ", "CSRS", "LPQ", "LPD", "LPG", "LPRP", "LSD", "LSQ", "LSRS", "RX", "ZTD", "ZTR", "GB", "YTD", "YTR"] ("Imp Type (0: CPD)")
            n264 = call "HP428XA Getting Started.vi"("Voltage Level (V) (1.0V)"=1.0, "Freq Value (Hz) (1.0 MHz)"="Freq Value (Hz) (500kHz)", "Imp Type (0: CPD)"=w803, "GPIB Address (15)"=w804) -> ("Secondary Value"=w801:dbl, "Primary Value"=w800:dbl)  [unwired: 4 in, 2 out]
            n265 = Wait (ms)(milliseconds to wait=u32 1000) -> ()  [unwired: 1 out]
          }
        }
        n266 = local read "Thickness"() -> (w798:dbl)
        n267 = local read "Area"() -> (w796:dbl)
        n268 = Multiply(x=w792, y=w798) -> (x*y=w797:dbl)
        n269 = Divide(x=w797, y=w796) -> (x/y=w795:dbl)
        n270 = Divide(x=w795, y=8.854e-12) -> (x/y=w788:dbl)
        "K500k" <- w788
        "C500k" <- w792
        "tand500k" <- w787
      }
      frame #14 {
        n271 = flat-sequence {
          tunnel: w833 -> [w851]
          tunnel: [w850] -> _
          tunnel: [w849] -> w831
          tunnel: w832 -> [w848]
          tunnel: [w848] -> w835
          frame #0 {
            n272 = call-poly "VISA Configure Serial Port"("VISA resource name"=w851, "data bits (8)"=7, "parity (0:none)"=1) -> ("error out"=w856:errorcluster)  [unwired: 11 in, 1 out]
            n273 = Concatenate Strings("*X01", "\r") -> (w859:string)
            n274 = VISA Write(VISA resource name=w851, write buffer=w859, error in (no error)=w856) -> (VISA resource name out=w870:refnum<visa-resource-name>, error out=w860:errorcluster)  [unwired: 1 out]
            n275 = property class="Instr"(reference=w870, error in=w860) -> (error out=w861:errorcluster, "Serial Settings:Number of Bytes at Serial Port"=w862:u32)  [unwired: 1 out]
            n276 = VISA Read(VISA resource name=w851, byte count=w862, error in (no error)=w861) -> (read buffer=w863:string, error out=w850:errorcluster)  [unwired: 2 out]
            n277 = String Length(string=w863) -> (length=w865:i32)
            n278 = Subtract(x=w865, y=4) -> (x-y=w867:i32)
            n279 = String Subset(string=w863, offset (0)=3, length (rest)=w867) -> (substring=w868:string)
            n280 = Concatenate Strings(w868, "\t") -> (w852:string)
            n281 = Scan Value(string=w852, format string="%f") -> (value=w849:dbl)  [unwired: 1 in, 1 out]
            "Temp1MHz" <- w849
          }
        }
        n282 = flat-sequence {
          tunnel: w835 -> [w846]
          tunnel: [w843] -> w829
          tunnel: [w842] -> w834
          frame #0 {
            w845 = u32 0 items=["CPD", "CPQ", "CPG", "CPRP", "CSD", "CSQ", "CSRS", "LPQ", "LPD", "LPG", "LPRP", "LSD", "LSQ", "LSRS", "RX", "ZTD", "ZTR", "GB", "YTD", "YTR"] ("Imp Type (0: CPD)")
            n283 = call "HP428XA Getting Started.vi"("Voltage Level (V) (1.0V)"=1.0, "Freq Value (Hz) (1.0 MHz)"="Freq Value (Hz) (1MHz)", "Imp Type (0: CPD)"=w845, "GPIB Address (15)"=w846) -> ("Secondary Value"=w843:dbl, "Primary Value"=w842:dbl)  [unwired: 4 in, 2 out]
            n284 = Wait (ms)(milliseconds to wait=u32 1000) -> ()  [unwired: 1 out]
          }
        }
        n285 = local read "Thickness"() -> (w840:dbl)
        n286 = local read "Area"() -> (w838:dbl)
        n287 = Multiply(x=w834, y=w840) -> (x*y=w839:dbl)
        n288 = Divide(x=w839, y=w838) -> (x/y=w837:dbl)
        n289 = Divide(x=w837, y=8.854e-12) -> (x/y=w830:dbl)
        "K1M" <- w830
        "C1M" <- w834
        "tand1M" <- w829
      }
    }
    n290 = flat-sequence {
      tunnel: w61 -> [w228]
      tunnel: w57 -> [w226]
      tunnel: w64 -> [w237]
      tunnel: w60 -> [w236]
      tunnel: w56 -> [w225]
      tunnel: w63 -> [w174]
      tunnel: w59 -> [w169]
      tunnel: w55 -> [w162]
      tunnel: w62 -> [w229]
      tunnel: w58 -> [w227]
      tunnel: w54 -> [w224]
      tunnel: w53 -> [w223]
      tunnel: w50 -> [w221]
      tunnel: w49 -> [w220]
      tunnel: w48 -> [w219]
      tunnel: w47 -> [w175]
      tunnel: w46 -> [w170]
      tunnel: w45 -> [w163]
      tunnel: w44 -> [w214]
      tunnel: w43 -> [w213]
      tunnel: w42 -> [w212]
      tunnel: w41 -> [w208]
      tunnel: w40 -> [w207]
      tunnel: w39 -> [w206]
      tunnel: w38 -> [w176]
      tunnel: w37 -> [w171]
      tunnel: w36 -> [w164]
      tunnel: w35 -> [w202]
      tunnel: w34 -> [w201]
      tunnel: w33 -> [w200]
      tunnel: w32 -> [w197]
      tunnel: w31 -> [w196]
      tunnel: w30 -> [w195]
      tunnel: w29 -> [w177]
      tunnel: w28 -> [w172]
      tunnel: w27 -> [w165]
      tunnel: w26 -> [w190]
      tunnel: w25 -> [w189]
      tunnel: w24 -> [w188]
      tunnel: w23 -> [w168]
      tunnel: w22 -> [w167]
      tunnel: w21 -> [w166]
      tunnel: w20 -> [w183]
      tunnel: w19 -> [w173]
      tunnel: w18 -> [w178]
      tunnel: [w168] -> w17
      tunnel: [w177] -> w16
      tunnel: [w176] -> w15
      tunnel: [w175] -> w14
      tunnel: [w174] -> w13
      tunnel: [w167] -> w12
      tunnel: [w172] -> w11
      tunnel: [w171] -> w10
      tunnel: [w170] -> w9
      tunnel: [w169] -> w8
      tunnel: [w166] -> w7
      tunnel: [w165] -> w6
      tunnel: [w164] -> w5
      tunnel: [w163] -> w4
      tunnel: [w162] -> w3
      frame #0 {
        w181 = 1000000000000.0 ("x")
        n291 = local read "C2.5k"() -> (w210:dbl)
        n292 = local read "C100k"() -> (w191:dbl)
        n293 = local read "C250k"() -> (w186:dbl)
        n294 = local read "C500k"() -> (w184:dbl)
        n295 = local read "C250"() -> (w217:dbl)
        n296 = local read "C10k"() -> (w203:dbl)
        n297 = local read "C25"() -> (w235:dbl)
        n298 = local read "C500"() -> (w222:dbl)
        n299 = local read "C25k"() -> (w198:dbl)
        n300 = local read "C100"() -> (w218:dbl)
        n301 = local read "C50k"() -> (w193:dbl)
        n302 = local read "C50"() -> (w230:dbl)
        n303 = local read "C1k"() -> (w215:dbl)
        n304 = local read "C5k"() -> (w205:dbl)
        n305 = local read "C1M"() -> (w180:dbl)
        n306 = Multiply(x=w181, y=w235) -> (x*y=w234:dbl)
        n307 = Multiply(x=w181, y=w230) -> (x*y=w233:dbl)
        n308 = Multiply(x=w181, y=w218) -> (x*y=w232:dbl)
        n309 = Multiply(x=w181, y=w222) -> (x*y=w216:dbl)
        n310 = Multiply(x=w181, y=w217) -> (x*y=w231:dbl)
        n311 = Multiply(x=w181, y=w215) -> (x*y=w211:dbl)
        n312 = Multiply(x=w181, y=w210) -> (x*y=w209:dbl)
        n313 = Multiply(x=w181, y=w205) -> (x*y=w204:dbl)
        n314 = Multiply(x=w181, y=w203) -> (x*y=w199:dbl)
        n315 = Multiply(x=w181, y=w198) -> (x*y=w194:dbl)
        n316 = Multiply(x=w181, y=w193) -> (x*y=w192:dbl)
        n317 = Multiply(x=w181, y=w191) -> (x*y=w187:dbl)
        n318 = Multiply(x=w181, y=w186) -> (x*y=w185:dbl)
        n319 = Multiply(x=w181, y=w184) -> (x*y=w182:dbl)
        n320 = Multiply(x=w181, y=w180) -> (x*y=w179:dbl)
        n321 = Build Array(w223, w234, w228, w226, w237, w233, w236, w225, w174, w232, w169, w162, w229, w231, w227, w224, w221, w216, w220, w219, w175, w211, w170, w163, w214, w209, w213, w212, w208, w204, w207, w206, w176, w199, w171, w164, w202, w194, w201, w200, w197, w192, w196, w195, w177, w187, w172, w165, w190, w185, w189, w188, w168, w182, w167, w166, w178, w179, w173, w183) -> (w240:dbl[])
        n322 = local read "Path & File Name (*.txt)"() -> (w238:path)
        n323 = call-poly <vilib>:"Write To Spreadsheet File.vi"("append to file? (new file:F)"=TRUE, "1D data"=w240, "file path (dialog if empty)"=w238) -> ()  [unwired: 5 in, 1 out]
      }
    }
    n324 = flat-sequence {
      tunnel: w13 -> [w128]
      tunnel: w14 -> [w127]
      tunnel: w15 -> [w126]
      tunnel: w16 -> [w125]
      tunnel: w8 -> [w124]
      tunnel: w9 -> [w123]
      tunnel: w10 -> [w122]
      tunnel: w11 -> [w121]
      tunnel: w3 -> [w120]
      tunnel: w4 -> [w119]
      tunnel: w5 -> [w118]
      tunnel: w6 -> [w117]
      tunnel: w17 -> [w81]
      tunnel: w12 -> [w73]
      tunnel: w7 -> [w66]
      frame #0 {
        n325 = Insert Into Array(array="Temp10k", index=0, new element=w126) -> (w88:dbl[])
        n326 = Insert Into Array(array="Temp500k", index=0, new element=w81) -> (w78:dbl[])
        n327 = Insert Into Array(array="Temp100", index=0, new element=w128) -> (w90:dbl[])
        n328 = Insert Into Array(array="Temp1k", index=0, new element=w127) -> (w89:dbl[])
        n329 = Insert Into Array(array="Temp100k", index=0, new element=w125) -> (w87:dbl[])
        n330 = Insert Into Array(array="K100", index=0, new element=w124) -> (w110:dbl[])
        n331 = Insert Into Array(array="K10k", index=0, new element=w122) -> (w108:dbl[])
        n332 = Insert Into Array(array="K500k", index=0, new element=w73) -> (w72:dbl[])
        n333 = Insert Into Array(array="K1k", index=0, new element=w123) -> (w109:dbl[])
        n334 = Insert Into Array(array="K100k", index=0, new element=w121) -> (w107:dbl[])
        n335 = Build Array(w89) -> (w104:dbl[][])
        n336 = Build Array(w88) -> (w102:dbl[][])
        n337 = Build Array(w87) -> (w100:dbl[][])
        n338 = Build Array(w78) -> (w83:dbl[][])
        n339 = Build Array(w90) -> (w106:dbl[][])
        n340 = call "Convert to Dynamic Data19"("Array"=w72) -> ("Dynamic Data Type"=w76:dynamicdata)  [unwired: 3 in]
        n341 = Build Array(w89) -> (w93:dbl[][])
        n342 = Build Array(w88) -> (w95:dbl[][])
        n343 = Build Array(w87) -> (w97:dbl[][])
        n344 = Build Array(w78) -> (w77:dbl[][])
        n345 = call "Convert to Dynamic Data5"("Array"=w110) -> ("Dynamic Data Type"=w116:dynamicdata)  [unwired: 3 in]
        n346 = call "Convert to Dynamic Data6"("Array"=w109) -> ("Dynamic Data Type"=w115:dynamicdata)  [unwired: 3 in]
        n347 = call "Convert to Dynamic Data7"("Array"=w108) -> ("Dynamic Data Type"=w114:dynamicdata)  [unwired: 3 in]
        n348 = call "Convert to Dynamic Data8"("Array"=w107) -> ("Dynamic Data Type"=w113:dynamicdata)  [unwired: 3 in]
        n349 = Build Array(w90) -> (w91:dbl[][])
        n350 = Insert Into Array(array="tand100", index=0, new element=w120) -> (w146:dbl[])
        n351 = Insert Into Array(array="tand1k", index=0, new element=w119) -> (w147:dbl[])
        n352 = Insert Into Array(array="tand10k", index=0, new element=w118) -> (w148:dbl[])
        n353 = Insert Into Array(array="tand100k", index=0, new element=w117) -> (w149:dbl[])
        n354 = Insert Into Array(array="tand500k", index=0, new element=w66) -> (w67:dbl[])
        n355 = call "Convert to Dynamic Data9"("Array"=w146) -> ("Dynamic Data Type"=w131:dynamicdata)  [unwired: 3 in]
        n356 = call "Convert to Dynamic Data10"("Array"=w147) -> ("Dynamic Data Type"=w132:dynamicdata)  [unwired: 3 in]
        n357 = call "Convert to Dynamic Data11"("Array"=w148) -> ("Dynamic Data Type"=w85:dynamicdata)  [unwired: 3 in]
        n358 = call "Convert to Dynamic Data12"("Array"=w149) -> ("Dynamic Data Type"=w71:dynamicdata)  [unwired: 3 in]
        n359 = call "Convert to Dynamic Data20"("Array"=w67) -> ("Dynamic Data Type"=w70:dynamicdata)  [unwired: 3 in]
        n360 = call "Convert to Dynamic Data13"("2D Array"=w106) -> ("Dynamic Data Type"=w105:dynamicdata)  [unwired: 3 in]
        n361 = call "Convert to Dynamic Data"("2D Array"=w104) -> ("Dynamic Data Type"=w103:dynamicdata)  [unwired: 3 in]
        n362 = call "Convert to Dynamic Data2"("2D Array"=w102) -> ("Dynamic Data Type"=w101:dynamicdata)  [unwired: 3 in]
        n363 = call "Convert to Dynamic Data3"("2D Array"=w100) -> ("Dynamic Data Type"=w99:dynamicdata)  [unwired: 3 in]
        n364 = call "Convert to Dynamic Data17"("2D Array"=w83) -> ("Dynamic Data Type"=w84:dynamicdata)  [unwired: 3 in]
        n365 = call "Convert to Dynamic Data4"("2D Array"=w91) -> ("Dynamic Data Type"=w92:dynamicdata)  [unwired: 3 in]
        n366 = call "Convert to Dynamic Data14"("2D Array"=w93) -> ("Dynamic Data Type"=w94:dynamicdata)  [unwired: 3 in]
        n367 = call "Convert to Dynamic Data15"("2D Array"=w95) -> ("Dynamic Data Type"=w96:dynamicdata)  [unwired: 3 in]
        n368 = call "Convert to Dynamic Data16"("2D Array"=w97) -> ("Dynamic Data Type"=w98:dynamicdata)  [unwired: 3 in]
        n369 = call "Convert to Dynamic Data18"("2D Array"=w77) -> ("Dynamic Data Type"=w79:dynamicdata)  [unwired: 3 in]
        n370 = Merge Signals(w105, w103, w101, w99, w84) -> (w111:dynamicdata)
        n371 = Merge Signals(w116, w115, w114, w113, w76) -> (w112:dynamicdata)
        n372 = Merge Signals(w92, w94, w96, w98, w79) -> (w86:dynamicdata)
        n373 = Merge Signals(w131, w132, w85, w71, w70) -> (w133:dynamicdata)
        n374 = call "Build XY Graph"("Y Input"=w112, "X Input"=w111) -> ("XY Graph"=→"Relative Permittivity vs. Temperature":cluster{"Y":dbl[], "Y":dbl[]}[])  [unwired: 8 in, 1 out]
        n375 = call "Build XY Graph2"("Y Input"=w133, "X Input"=w86) -> ("XY Graph"=→"Dielectric Loss vs. Temperature":cluster{"Y":dbl[], "Y":dbl[]}[])  [unwired: 8 in, 1 out]
      }
    }
  }
  n376 = while {
    tunnel: ["Path & File Name (*.txt)"] -> w2
    stop <- "Run" stop-if-true
    n377 = Multiply(x="Diameter (mm)", y=0.001) -> (x*y=w879:dbl)
    n378 = Divide(x=w879, y=2) -> (x/y=w874:dbl)
    n379 = Wait (ms)(milliseconds to wait=u32 100) -> ()  [unwired: 1 out]
    n380 = Square(x=w874) -> (x^2=w875:dbl)
    n381 = Multiply(x="Thickness (mm)", y=0.001) -> (x*y=→"Thickness":dbl)
    n382 = Multiply(x=3.141592653589793, y=w875) -> (x*y=→"Area":dbl)
  }
  n383 = flat-sequence {
    tunnel: w2 -> [w946]
    tunnel: [w944] -> w1
    frame #0 {
      w913 = "\t"
      w914 = "Temperature (C)" ("string")
      n384 = local read "Thickness"() -> (w950:dbl)
      n385 = local read "Area"() -> (w951:dbl)
      n386 = Number To Exponential String(number=w951) -> (E-format string=w943:string)  [unwired: 3 in]
      n387 = Number To Exponential String(number=w950) -> (E-format string=w941:string)  [unwired: 3 in]
      n388 = Concatenate Strings("Thickness (m)" ("string"), "\t", w941) -> (w939:string)
      n389 = Concatenate Strings("Area (m^2)" ("string"), "\t", w943) -> (w947:string)
      n390 = Concatenate Strings("Comment" ("string"), "\t", "Comment (Sample's Name, compositions, whatever you want,..)", "\r", w947, "\t", w939, "\r", w914, w913, "C25Hz (pF)" ("string"), w913, "K25Hz" ("string"), w913, "tand25Hz" ("string"), w913, w914, w913, "C50Hz (pF)" ("string"), w913, "K50Hz" ("string"), w913, "tand50Hz" ("string"), w913, w914, w913, "C100Hz (pF)" ("string"), w913, "K100Hz" ("string"), w913, "tand100Hz" ("string"), w913, w914, w913, "C250Hz (pF)" ("string"), w913, "K250Hz" ("string"), w913, "tand250Hz" ("string"), w913, w914, w913, "C500Hz (pF)" ("string"), w913, "K500Hz" ("string"), w913, "tand500Hz" ("string"), w913, w914, w913, "C1kHz (pF)" ("string"), w913, "K1kHz" ("string"), w913, "tand1kHz" ("string"), w913, w914, w913, "C2.5kHz (pF)" ("string"), w913, "K2.5kHz" ("string"), w913, "tand2.5kHz" ("string"), w913, w914, w913, "C5kHz (pF)" ("string"), w913, "K5kHz" ("string"), w913, "tand5kHz" ("string"), w913, w914, w913, "C10kHz (pF)" ("string"), w913, "K10kHz" ("string"), w913, "tand10kHz" ("string"), w913, w914, w913, "C25kHz (pF)" ("string"), w913, "K25kHz" ("string"), w913, "tand25kHz" ("string"), w913, w914, w913, "C50kHz (pF)" ("string"), w913, "K50kHz" ("string"), w913, "tand50kHz" ("string"), w913, w914, w913, "C100kHz (pF)" ("string"), w913, "K100kHz" ("string"), w913, "tand100kHz" ("string"), w913, w914, w913, "C250kHz (pF)" ("string"), w913, "K250kHz" ("string"), w913, "tand250kHz" ("string"), w913, w914, w913, "C500kHz (pF)" ("string"), w913, "K500kHz" ("string"), w913, "tand500kHz" ("string"), w913, w914, w913, "C1MHz (pF)" ("string"), w913, "K1MHz" ("string"), w913, "tand1MHz" ("string"), "\r\n") -> (w945:string)
      n391 = Write to Text File(file (use dialog)=w946, text=w945) -> (error out=w944:errorcluster)  [unwired: 2 in, 2 out]
    }
  }
